vi "test6-Interrupt_Queue.vi"(8 "error in (no error)":errorcluster, 11 "TestCase in":refnum<class "testcase-CSMGlobalLog.lvclass">) -> (0 "error out":errorcluster, 3 "TestCase out":refnum<class "testcase-CSMGlobalLog.lvclass">)   [LabVIEW 2017, in "testcase-CSMGlobalLog.lvclass"]
uses:
  testcase-CSMGlobalLog.lvclass
  testcase-CSMGlobalLog.lvclass/testcase-CSMGlobalLog.ctl
  f2908a69-50b3-4358-8c93-3e573ca7d2ca.vi
  <vilib>/addons/_JKI Toolkits/VI Tester/TestCase.llb/TestCase.lvclass
  src/user.lib/_NEVSTOP/Communicable State Machine(CSM)/Communicable State Machine.lvlib
  src/user.lib/_NEVSTOP/Communicable State Machine(CSM)/Utility/Periodic String Filter Setting.ctl
  C:/Program Files (x86)/National Instruments/LabVIEW 2017/vi.lib/addons/_JKI Toolkits/VI Tester/TestCase.llb/TestCase.lvclass
panel:
  out "String cache total":string
  out "error out 3":errorcluster
  out "LoopCount":i32
  out "String Cache Each Loop":string
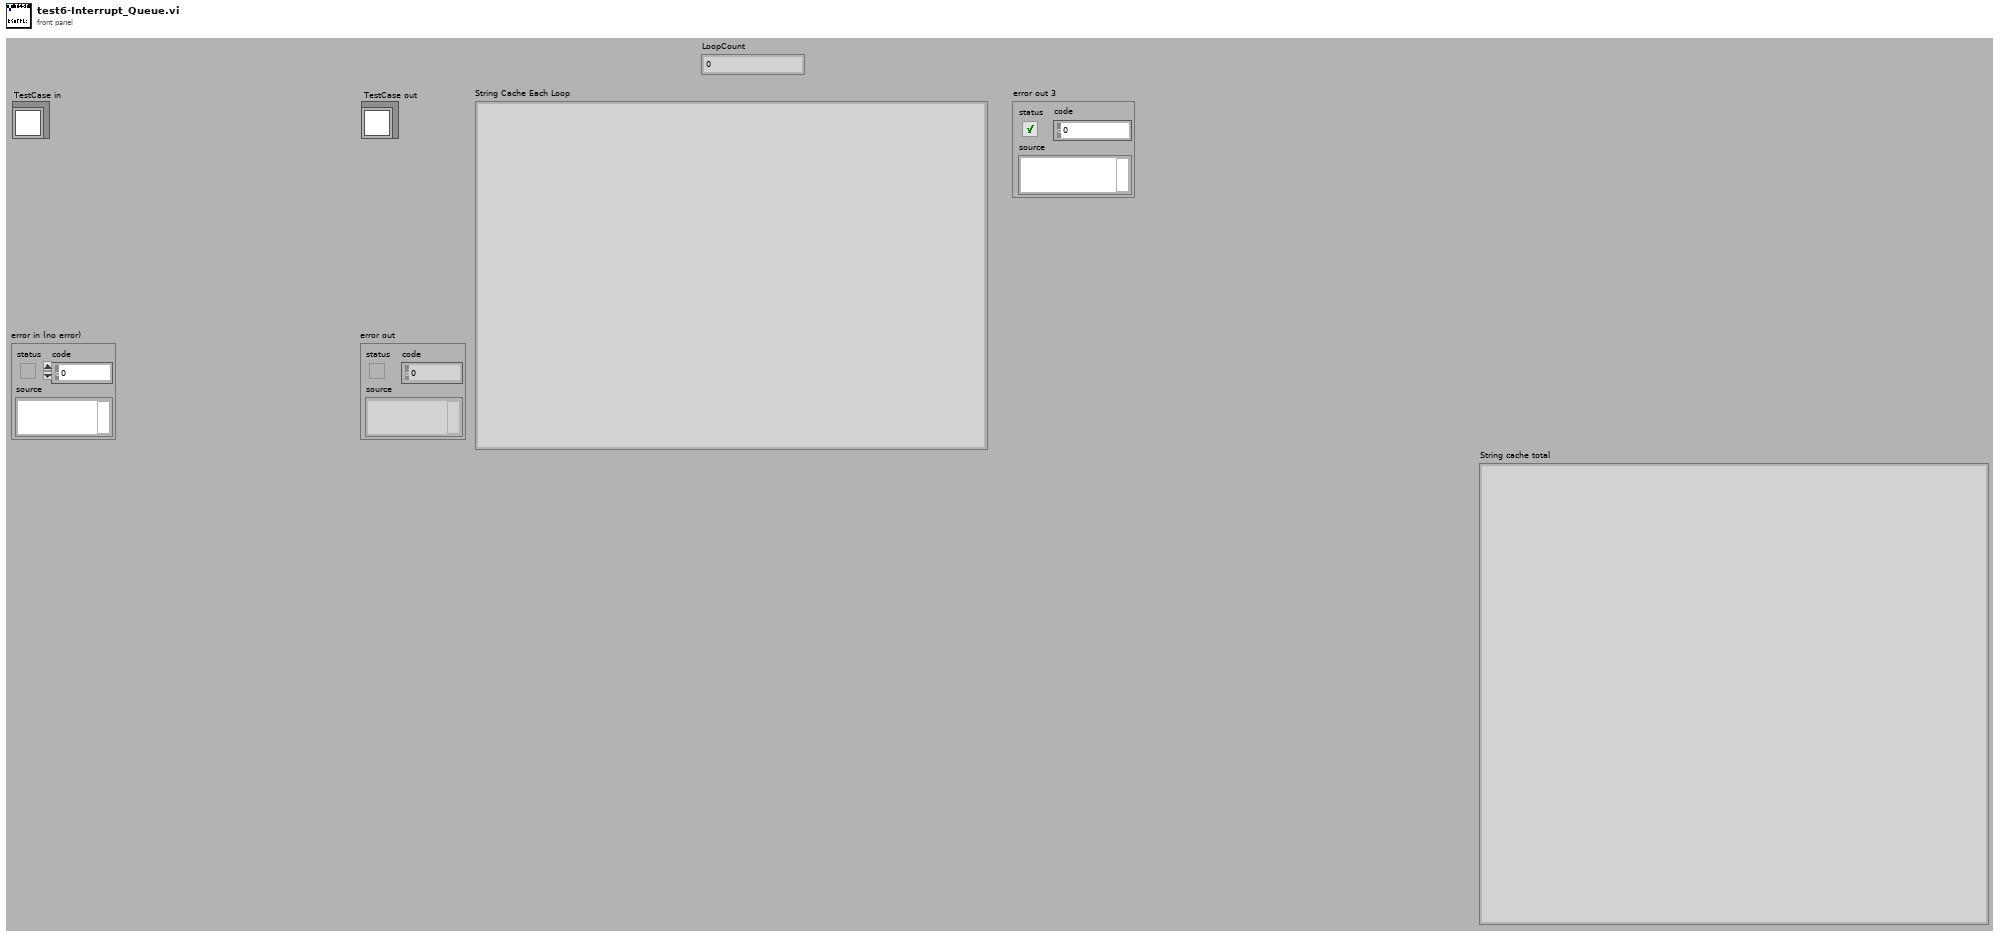
[diagram p1: front panel]
types:
  T1 = typedef "Communicable State Machine.lvlib/Periodic String Filter Setting.ctl" = cluster{"threashold(#/s)":dbl, "Check Peroid(s)":dbl}
  T2 = typedef "Communicable State Machine.lvlib/_CSM_GlobalLog_MSG.ctl" = cluster{"Name (\"\" to Use UUID)":string, "Current State":string, "Arguments":string, "Source Message":T3, "Source Module":string, "Complete(T)/Start(F)":bool, "LogType":T4, "Time Stamp":timestamp}
  T3 = typedef "Communicable State Machine.lvlib/_CSM_Response Source Message.ctl" = cluster{"‘State":string, "’Arguments":string, "’Error":errorcluster}
  T4 = typedef "Communicable State Machine.lvlib/_CSM_GlobalLog_MSG_TYPE.ctl" = enum16{"User Log", "State Change", "Status", "Interrupt", "Register", "Unregister", "Error Log", "Module Created", "Module Destroyed"}
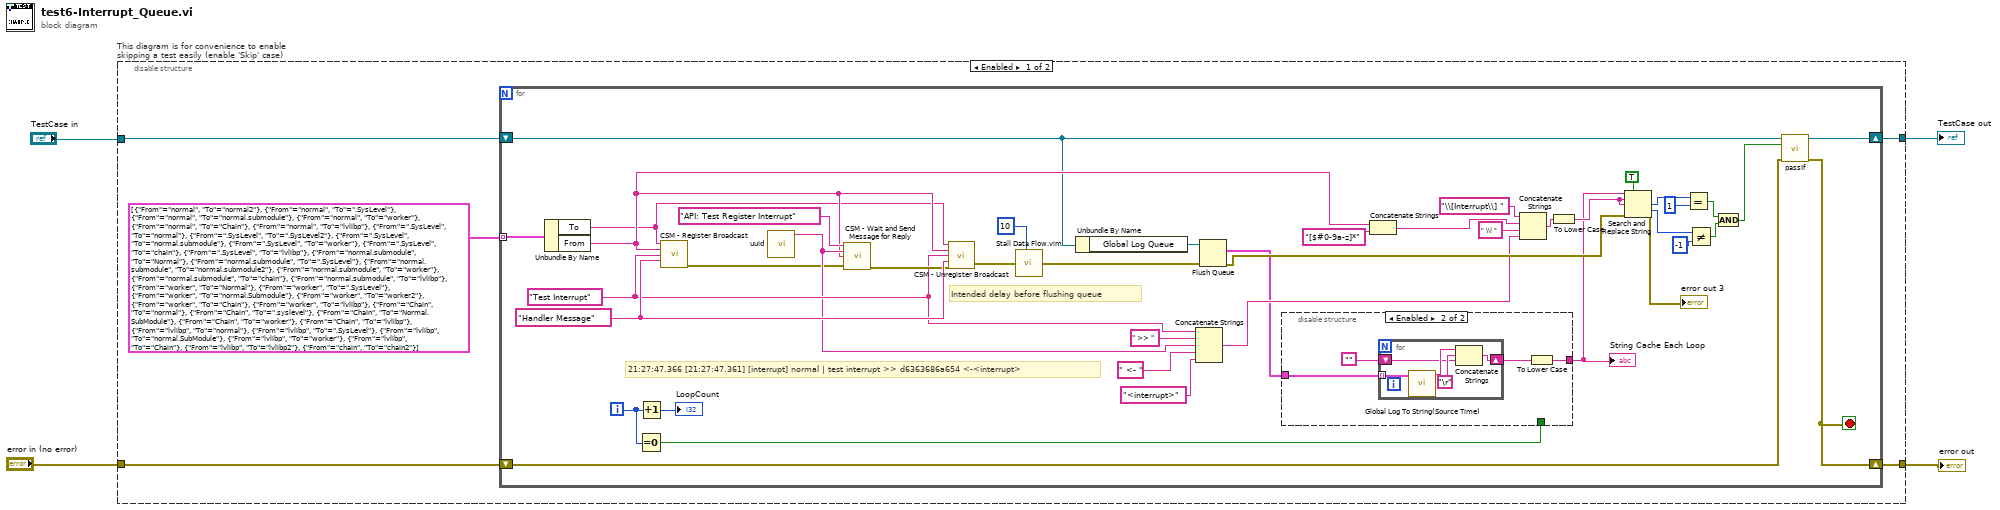
[diagram p0: block diagram]
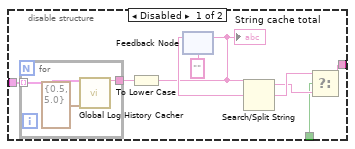
[diagram p2: hidden frame]
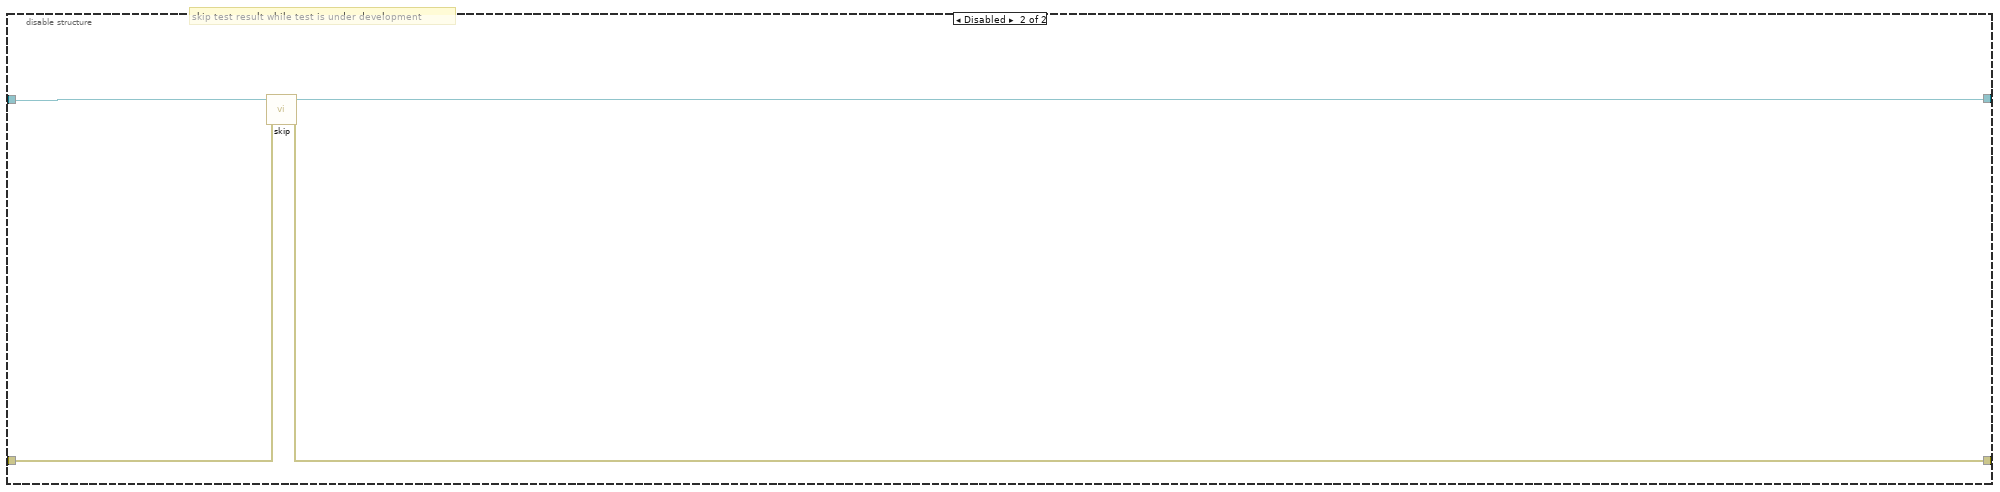
[diagram p3: hidden frame]
diagram:
  n1 = disable-structure "This diagram is for convenience to enable skipping a test easily (enable 'Skip' case)" shown="Enabled" {
    disable-tunnel: "TestCase in" -> [w5 w76]
    disable-tunnel: [w8 w74] -> w1
    disable-tunnel: [w9 w75] -> w3
    disable-tunnel: "error in (no error)" -> [w7 w73]
    frame Enabled {
      n2 = for {
        tunnel: cluster{"From":string, "To":string}[] [{"From"="normal", "To"="normal2"}, {"From"="normal", "To"=".SysLevel"}, {"From"="normal", "To"="normal.submodule"}, {"From"="normal", "To"="worker"}, {"From"="normal", "To"="Chain"}, {"From"="normal", "To"="lvlibp"}, {"From"=".SysLevel", "To"="normal"}, {"From"=".SysLevel", "To"=".SysLevel2"}, {"From"=".SysLevel", "To"="normal.submodule"}, {"From"=".SysLevel", "To"="worker"}, {"From"=".SysLevel", "To"="chain"}, {"From"=".SysLevel", "To"="lvlibp"}, {"From"="normal.submodule", "To"="Normal"}, {"From"="normal.submodule", "To"=".SysLevel"}, {"From"="normal.submodule", "To"="normal.submodule2"}, {"From"="normal.submodule", "To"="worker"}, {"From"="normal.submodule", "To"="chain"}, {"From"="normal.submodule", "To"="lvlibp"}, {"From"="worker", "To"="Normal"}, {"From"="worker", "To"=".SysLevel"}, {"From"="worker", "To"="normal.Submodule"}, {"From"="worker", "To"="worker2"}, {"From"="worker", "To"="Chain"}, {"From"="worker", "To"="lvlibp"}, {"From"="Chain", "To"="normal"}, {"From"="Chain", "To"=".syslevel"}, {"From"="Chain", "To"="Normal.SubModule"}, {"From"="Chain", "To"="worker"}, {"From"="Chain", "To"="lvlibp"}, {"From"="lvlibp", "To"="normal"}, {"From"="lvlibp", "To"=".SysLevel"}, {"From"="lvlibp", "To"="normal.SubModule"}, {"From"="lvlibp", "To"="worker"}, {"From"="lvlibp", "To"="Chain"}, {"From"="lvlibp", "To"="lvlibp2"}, {"From"="chain", "To"="chain2"}] -> [w38] mode=indexing
        shift-right: [w19] -> w9
        shift-left: w7 -> [w49]
        shift-right: [w51] -> w8
        shift-left: w5 -> [w21]
        i -> [w12]
        stop <- w19 stop-if-true
        w37 = "Handler Message" ("API (If \"\", Same as Trigger)")
        w30 = "Test Interrupt" ("Trigger")
        # "Intended delay before flushing queue"
        # "21:27:47.366 [21:27:47.361] [interrupt] normal | test interrupt >> d6363686a654 <-<interrupt>"
        n3 = Unbundle By Name(w38) -> ("To"=w10:string, "From"=w24:string)
        n4 = Equal To 0?(x=w12) -> (x = 0?=w11:bool)
        n5 = Increment(x=w12) -> (x+1=→"LoopCount":i32)
        n6 = call "CSM - Register Broadcast.vi"("CSM Name"=w10, "Source CSM Name (* as Default)"=w24, "Trigger"=w30, "API (If \"\", Same as Trigger)"=w37) -> ("error out"=w20:errorcluster)  [unwired: 10 in, 1 out]
        n7 = call "uuid.vi"() -> ("UUID"=w28:string)  [unwired: 11 in]
        n8 = call "CSM - Wait and Send Message for Reply.vi"("State"="API: Test Register Interrupt", "Arguments (\"\")"=w28, "Target Module"=w24, "Error In (No Error)"=w20) -> ("error out"=w35:errorcluster)  [unwired: 9 in, 2 out]
        n9 = call "CSM - Unregister Broadcast.vi"("CSM Name"=w10, "Source CSM Name (* as Default)"=w24, "Trigger"=w30, "API (\"*\" as Default)"=w37, "Error In"=w35) -> ("error out"=w17:errorcluster)  [unwired: 9 in, 1 out]
        n10 = call "Stall Data Flow.vim"("value in"=w17, "milliseconds to wait"=u32 10 ("millisecond timer value")) -> ("value out"=w16:errorcluster)  [unwired: 1 out]
        n11 = Unbundle By Name(w21) -> ("Global Log Queue"=w50:refnum<queue>)
        n12 = Concatenate Strings(w30, " >> " ("string"), w28, " <- " ("string"), "<interrupt>" ("search string")) -> (w26:string)
        n13 = Flush Queue(queue=w50, error in (no error)=w16) -> (remaining elements=w13:T2[], error out=w40:errorcluster)  [unwired: 1 out]
        n14 = disable-structure shown="Enabled" {
          disable-tunnel: [w54 w64] -> w14
          disable-tunnel: w11 -> [w53 _]
          disable-tunnel: w13 -> [w52 w66]
          frame Disabled {
            n15 = for {
              tunnel: w52 -> [w63] mode=indexing
              tunnel: [w62] -> w60
              n16 = call "Global Log History Cacher.vi"("Global Log Data"=w63, "Settings"=T1 {"threashold(#/s)"=0.5, "Check Peroid(s)"=5.0}) -> ("String Cache"=w62:string)  [unwired: 13 in]
            }
            n17 = To Lower Case(string=w60) -> (all lower case string=w55:string)
            "String cache total" <- w55
            n18 = feedback #1("") -> (w59:string)
            n19 = feedback-in #1(w55) -> ()
            n20 = Search/Split String(string=w55, search string/char (-)=w59) -> (substring before match=w56:string, match + rest of string=w57:string)  [unwired: 1 in, 1 out]
            n21 = Select(t=w57, s=w53, f=w56) -> (s? t:f=w54:string)
          }
          frame Enabled {
            n22 = for {
              tunnel: w66 -> [w72] mode=indexing
              shift-right: [w68] -> w65
              shift-left: "" -> [w69]
              n23 = call "Global Log To String(Source Time).vi"("Log"=w72) -> ("Log String"=w71:string)  [unwired: 9 in]
              n24 = Concatenate Strings(w71, "\r", w69) -> (w68:string)
            }
            n25 = To Lower Case(string=w65) -> (all lower case string=w64:string)
          }
        }
        "String Cache Each Loop" <- w14
        n26 = Concatenate Strings(w24, "[$#0-9a-z]*" ("string")) -> (w22:string)
        n27 = Concatenate Strings("\\[Interrupt\\] " ("regular expression"), w22, " \\| " ("string"), w26) -> (w33:string)
        n28 = To Lower Case(string=w33) -> (all lower case string=w46:string)
        n29 = Search and Replace String(replace all?=TRUE ("replace all? (F)"), input string=w14, search string=w46, replace string=w46, error in=w40) -> (number of replacements=w45:i32, offset past replacement=w44:i32, error out=→"error out 3":errorcluster)  [unwired: 3 in, 1 out]
        n30 = Equal?(x=w45, y=1) -> (x = y?=w42:bool)
        n31 = Not Equal?(x=w44, y=-1) -> (x != y?=w41:bool)
        n32 = And(x=w42, y=w41) -> (x .and. y?=w18:bool)
        n33 = call-dynamic "passIf.vi"("error in (no error)"=w49, "pass"=w18, "TestCase in"=w21) -> ("error out"=w19:errorcluster, "TestCase out"=w51:refnum<class "testcase-CSMGlobalLog.lvclass">)  [unwired: 7 in]
      }
    }
    frame Disabled {
      # "skip test result while test is under development"
      n34 = call <vilib>:"skip.vi"("error in (no error)"=w73, "TestCase in"=w76) -> ("error out"=w75:errorcluster, "TestCase out"=w74:refnum<class "testcase-CSMGlobalLog.lvclass">)  [unwired: 8 in]
    }
  }
  "error out" <- w3
  "TestCase out" <- w1
